vi "GOMDBTS2048 weighting Get Available Funtions.vi"(8 "error in (no error)":errorcluster, 11 "handle":i32) -> (0 "error out":errorcluster, 1 "identifiers and names":cluster{"identifiers":i32, "names":string}[](array[cluster]), 2 "function return":i32, 3 "quantity":i32)   [LabVIEW 2015, in "GOMDBTS2048.lvlib"]
doc: "GOBTS2048DLL int __stdcall GOMDBTS2048_integralGetWeightingFactors(int handle, int parameter, double* value);"
uses:
  GOMDBTS2048.lvlib
  runtime/GOMDBTS2048.dll
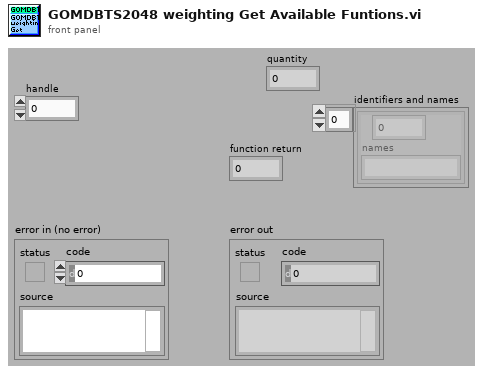
[diagram p1: front panel]
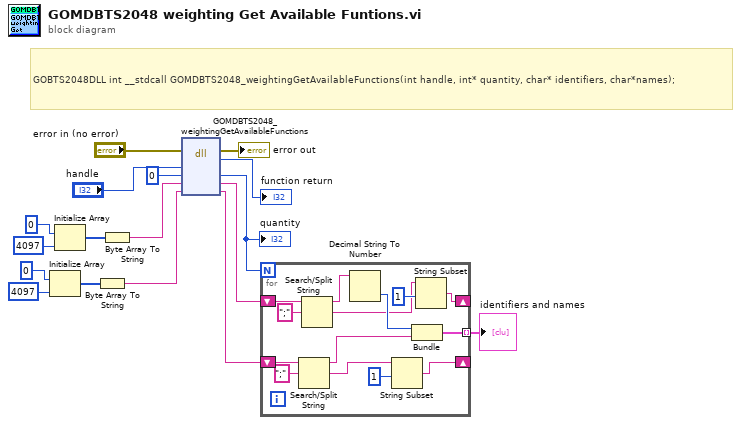
[diagram p0: block diagram]
diagram:
  # "GOBTS2048DLL int __stdcall GOMDBTS2048_weightingGetAvailableFunctions(int handle, int* quantity, char* identifiers, char*names);"
  n1 = Initialize Array(u8 0 ("element"), 4097 ("dimension size")) -> (w8:u8[])
  n2 = Initialize Array(u8 0 ("element"), 4097 ("dimension size")) -> (w11:u8[])
  n3 = Byte Array To String(unsigned byte array=w8) -> (string=w5:string)
  n4 = Byte Array To String(unsigned byte array=w11) -> (string=w9:string)
  n5 = dll-call lib="C:/Users/rkoch/Documents/GO_Library/runtime/GOMDBTS2048.*" fn="GOMDBTS2048_weightingGetAvailableFunctions"(error in="error in (no error)", "handle"="handle", "quantity"=0, "identifiers"=w9, "names"=w5) -> (error out=→"error out":errorcluster, "return type"=→"function return":i32, "quantity"=w4:i32, "identifiers"=w3:string, "names"=w2:string)  [unwired: 3 in, 1 out]
  "quantity" <- w4
  n6 = for {
    N: w4 -> [_]
    shift-right: [w18] -> _
    shift-left: w3 -> [w31]
    shift-right: [w21] -> _
    shift-left: w2 -> [w28]
    tunnel: [w24] -> w1 mode=indexing
    n7 = Search/Split String(string=w28, search string/char (-)=";") -> (substring before match=w25:string, match + rest of string=w22:string)  [unwired: 1 in, 1 out]
    n8 = Search/Split String(string=w31, search string/char (-)=";") -> (substring before match=w27:string, match + rest of string=w19:string)  [unwired: 1 in, 1 out]
    n9 = Decimal String To Number(string=w27) -> (number=w26:i32)  [unwired: 2 in, 1 out]
    n10 = String Subset(string=w22, offset (0)=1) -> (substring=w21:string)  [unwired: 1 in]
    n11 = Bundle(w26, "names"=w25) -> (w24:cluster{i32, "names":string})  [unwired: 1 in]
    n12 = String Subset(string=w19, offset (0)=1) -> (substring=w18:string)  [unwired: 1 in]
  }
  "identifiers and names" <- w1
